vi "Init Xnet CAN.vi"(8 "error in":errorcluster, 10 "XNET Communication Properties In":T1 {"CAN I/O Mode" items=["CAN", "CAN FD", "CAN FD + BRS"]}, 11 "ForceInitAsSubordinate":bool) -> (0 "error out":errorcluster {"code" format="%.0x"}, 2 "XNET Communication Properties Out":T1 {"CAN I/O Mode" items=["CAN", "CAN FD", "CAN FD + BRS"]}, 3 "Init Stat":bool)   [LabVIEW 2014, in "CAN Bus Monitor Engine.lvlib"]
uses:
  CAN Bus Monitor Engine.lvlib
  Controls/XNET Communication Properties.ctl
  Controls/CAN IO Mode.ctl
  <vilib>/xnet/xnet.llb/XNET Create Session (Frame Input Stream).vi
  BM Global Vars.vi
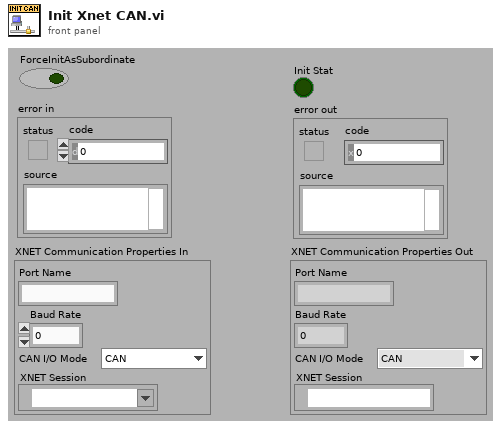
[diagram p1: front panel]
types:
  T1 = typedef "CAN Bus Monitor Engine.lvlib/XNET Communication Properties.ctl" = cluster{"Port Name":string, "Baud Rate":u32, "CAN I/O Mode":T2, "XNET Session":refnum<k21>}
  T2 = typedef "CAN Bus Monitor Engine.lvlib/CAN IO Mode.ctl" = u32
  T3 = cluster{"IncMinFrameTime":dbl, "IncMaxFrameTime":dbl, "Min Frame Length":dbl[][], "Max Frame Length":dbl[][], "Std Frames":u32, "Ext Frames":u32, "Error Frames":u32, "Remote Frames":u32, "Std Frames / Sec":u32, "Ext Frames / Sec":u32, "Error Frames / Sec":u32, "Remote Frames / Sec":u32, "Peak Bus Load":dbl, "Bus Load":dbl, "Start Timestamp":dbl, "Null Frames":u32, "Null Frames / Sec":u32}
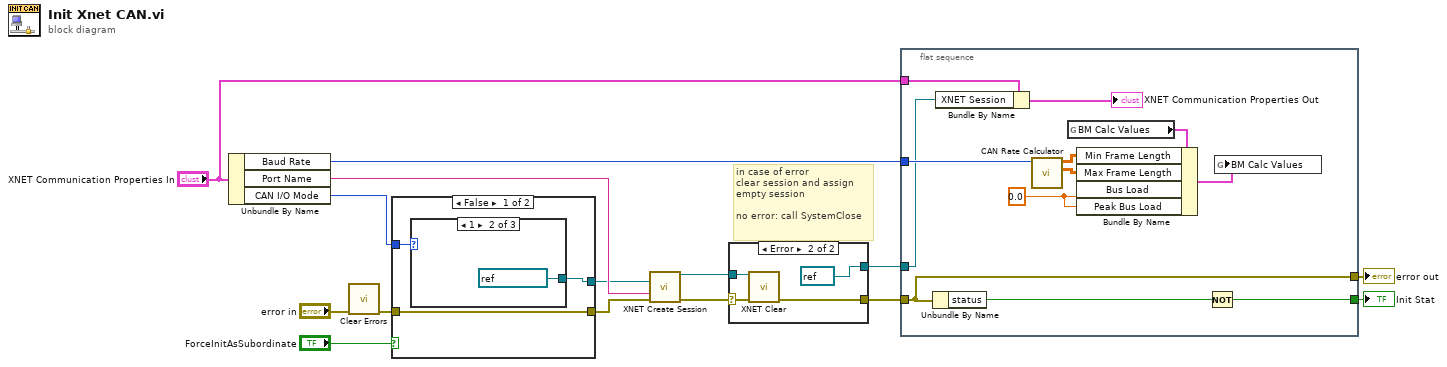
[diagram p0: block diagram]
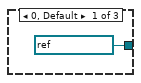
[diagram p2: hidden frame]
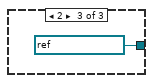
[diagram p3: hidden frame]
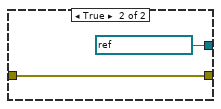
[diagram p4: hidden frame]
diagram:
  # "in case of error\nclear session and assign\nempty session\n\nno error: call SystemClose"
  n1 = Unbundle By Name("XNET Communication Properties In") -> ("Baud Rate"=w10:u32, "Port Name"=w13:string, "CAN I/O Mode"=w7:T2)
  n2 = call <vilib>:"Clear Errors.vi"("error in (no error)"="error in") -> ("error out"=w8:errorcluster)  [unwired: 5 in, 1 out]
  n3 = case shown="False" "ForceInitAsSubordinate" {
    tunnel: w8 -> [w18 w23]
    tunnel: [w18 w23] -> w6
    tunnel: [w16 refnum<k21> ":subordinate:" ("cluster (:memory:)")] -> w5
    tunnel: w7 -> [w17 _]
    frame False {
      n4 = case shown="1" w17 {
        tunnel: [refnum<k21> ":memory:" ("cluster (:memory:)") refnum<k21> ":can_fd:" ("cluster (:memory:)") refnum<k21> ":can_fd_brs:" ("cluster (:memory:)")] -> w16
        frame 0, Default {
        }
        frame 1 {
        }
        frame 2 {
        }
      }
    }
    frame True {
    }
  }
  n5 = call-poly <vilib>:"XNET Create Session.vi"("cluster (:memory:)"=w5, "interface"=w13, "error in (no error)"=w6) -> ("session out"=w4:refnum<k21>, "error out"=w3:errorcluster)  [unwired: 11 in]
  n6 = case shown="Error" w3 {
    selector: w3 -> [w24 w26]
    tunnel: w4 -> [w25 w29]
    tunnel: [w24 w27] -> w11
    tunnel: [w25 refnum<k21> refnum ("session out")] -> w12
    frame No Error {
    }
    frame Error {
      n7 = call <vilib>:"XNET Clear.vi"("session in"=w29, "error in (no error)"=w26) -> ("error out"=w27:errorcluster)  [unwired: 13 in]
    }
  }
  n8 = flat-sequence {
    tunnel: w11 -> [w34]
    tunnel: w12 -> [w32]
    tunnel: w10 -> [w39]
    tunnel: [w34] -> w15
    tunnel: [w35] -> w14
    tunnel: "XNET Communication Properties In" -> [w33]
    frame #0 {
      w30 = 0.0 ("Bus Load")
      n9 = Unbundle By Name(w34) -> ("status"=w36:bool)
      n10 = Bundle By Name(cluster=w33, "XNET Session"=w32) -> (→"XNET Communication Properties Out":T1)
      n11 = call "CAN Rate Calculator.vi"("Baud Rate"=w39) -> ("Max Frame Length"=w37:dbl[][], "Min Frame Length"=w38:dbl[][])  [unwired: 9 in]
      n12 = global read "BM Global Vars.vi" "BM Calc Values"() -> (w41:T3)
      n13 = Bundle By Name(cluster=w41, "Min Frame Length"=w38, "Max Frame Length"=w37, "Bus Load"=w30, "Peak Bus Load"=w30) -> (w40:T3)
      n14 = Not(x=w36) -> (.not. x?=w35:bool)
      n15 = global write "BM Global Vars.vi" "BM Calc Values"(w40) -> ()
    }
  }
  "error out" <- w15
  "Init Stat" <- w14
